vi "getK_p.vi"(11 "PIDController in":refnum<class "PIDController.lvclass">) -> (2 "k_p":dbl, 3 "PIDController out":refnum<class "PIDController.lvclass">)   [LabVIEW 2025, in "PIDController.lvclass"]
uses:
  PIDController.lvclass
  PIDController.lvclass/PIDController.ctl
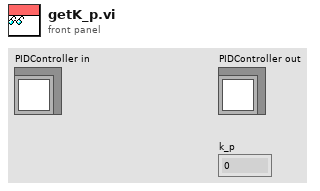
[diagram p1: front panel]
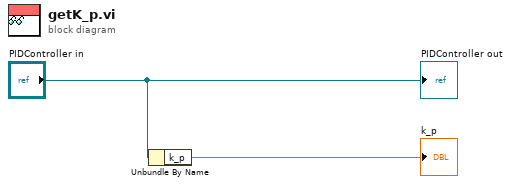
[diagram p0: block diagram]
diagram:
  n1 = Unbundle By Name("PIDController in") -> ("k_p"=→"k_p":dbl)
  "PIDController out" <- "PIDController in"
